vi "SENS_FOM_RANGE_SEGM_POWER_CONTROL.vi"(0 "VISA IN":refnum<visa-resource-name>, 1 "Range":i32, 2 "Enable Power Level? ON/OFF":bool, 5 "error in":errorcluster, 7 "Channel":i32) -> (14 "VISA Out":refnum<visa-resource-name>, 19 "error out":errorcluster)   [LabVIEW 2018, in "PNA-X.lvlib"]
uses:
  PNA-X.lvlib
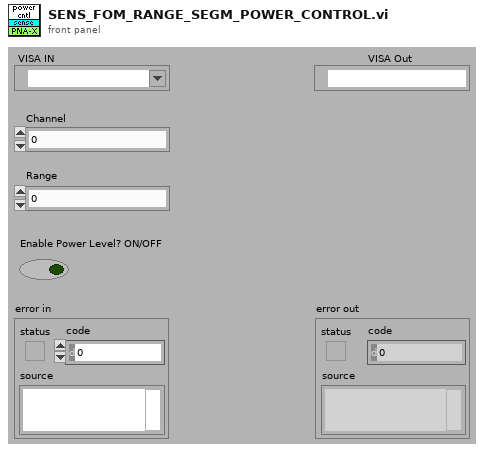
[diagram p1: front panel]
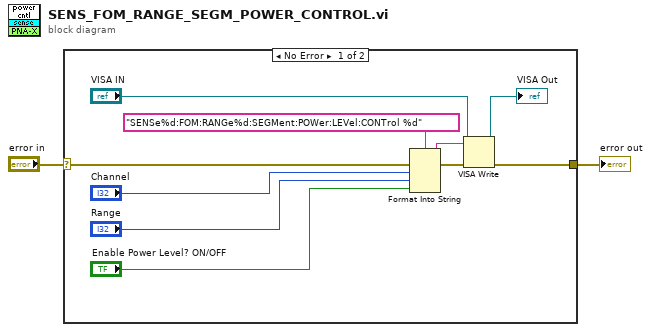
[diagram p0: block diagram]
diagram:
  n1 = case shown="No Error" "error in" {
    selector: "error in" -> [w12 w13]
    tunnel: [w7 w13] -> w1
    frame No Error {
      n2 = Format Into String(format string="SENSe%d:FOM:RANGe%d:SEGMent:POWer:LEVel:CONTrol %d" ("Cmdline"), error in=w12, "Channel", "Range", "Enable Power Level? ON/OFF") -> (resulting string=w10:string, error out=w11:errorcluster)  [unwired: 1 in]
      n3 = VISA Write(VISA resource name="VISA IN", write buffer=w10, error in (no error)=w11) -> (VISA resource name out=→"VISA Out":refnum<visa-resource-name>, error out=w7:errorcluster)  [unwired: 1 out]
    }
    frame Error {
    }
  }
  "error out" <- w1
